vi "Simulator PWM Measure.vi"(7 "PWM Stimulus":T1, 8 "error in (no error)":errorcluster, 10 "Target Value":dbl) -> (0 "error out":errorcluster {"code" format="%.0x"}, 2 "PWM Measurement":T2 caption="This reading is allways in the base units\ni.e. V, A, Ohms, Hz, Sec, etc." format="%#_10f")   [LabVIEW 2011]
uses:
  PWM Measurement.ctl
  PWM Parameters.ctl
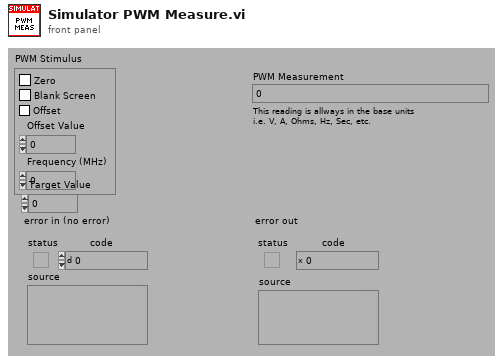
[diagram p1: front panel]
types:
  T1 = typedef "PWM Parameters.ctl" = cluster{"Zero":bool, "Blank Screen":bool, "Offset":bool, "Offset Value":dbl, "Frequency (MHz)":dbl}
  T2 = typedef "PWM Measurement.ctl" = dbl
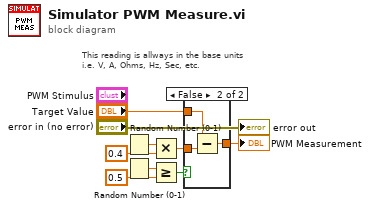
[diagram p0: block diagram]
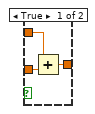
[diagram p2: hidden frame]
diagram:
  # "This reading is allways in the base units\ni.e. V, A, Ohms, Hz, Sec, etc."
  n1 = Random Number (0-1)() -> (number: 0 to 1=w9:dbl)
  n2 = Random Number (0-1)() -> (number: 0 to 1=w6:dbl)
  n3 = Multiply(x=w9, y=0.4) -> (x*y=w2:dbl)
  n4 = Greater Or Equal?(x=w6, y=0.5) -> (x >= y?=w4:bool)
  n5 = case shown="False" w4 {
    tunnel: "Target Value" -> [w10 w14]
    tunnel: w2 -> [w11 w13]
    tunnel: [w12 w15] -> w1
    frame True {
      n6 = Add(x=w10, y=w11) -> (x+y=w12:dbl)
    }
    frame False {
      n7 = Subtract(x=w14, y=w13) -> (x-y=w15:dbl)
    }
  }
  "PWM Measurement" <- w1
  "error out" <- "error in (no error)"
